vi "ReverseNot.vi"(4 "In":bool) -> (0 "~In":bool)   [LabVIEW 2012]
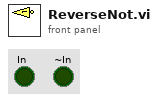
[diagram p1: front panel]
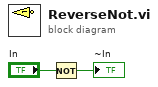
[diagram p0: block diagram]
diagram:
  n1 = Not(x="In") -> (.not. x?=→"~In":bool)
